vi "SomethingWith-FM.vi"() -> ()   [LabVIEW 2013]
uses:
  <vilib>/gmath/NI_Gmath.lvlib
panel:
  in  "N":dbl=1.0 caption="Numero de ciclos" format="%#_13g"
  out "mod":cluster{dbl[], dbl[]}(graph) caption="Modulação"
  out "Portadora":cluster{dbl[], dbl[]}(graph)
  out "Informação":cluster{dbl[], dbl[]}(graph)
  in  "Nc":dbl caption="Numero de amostras"
  in  "fm":dbl caption="Frequencia do sinal modulador"
  in  "fp":dbl caption="Frequencia da portadora"
  in  "E0":dbl caption="Amplitude da portadora"
  in  "Em":dbl caption="Amplitude do sinal modulador"
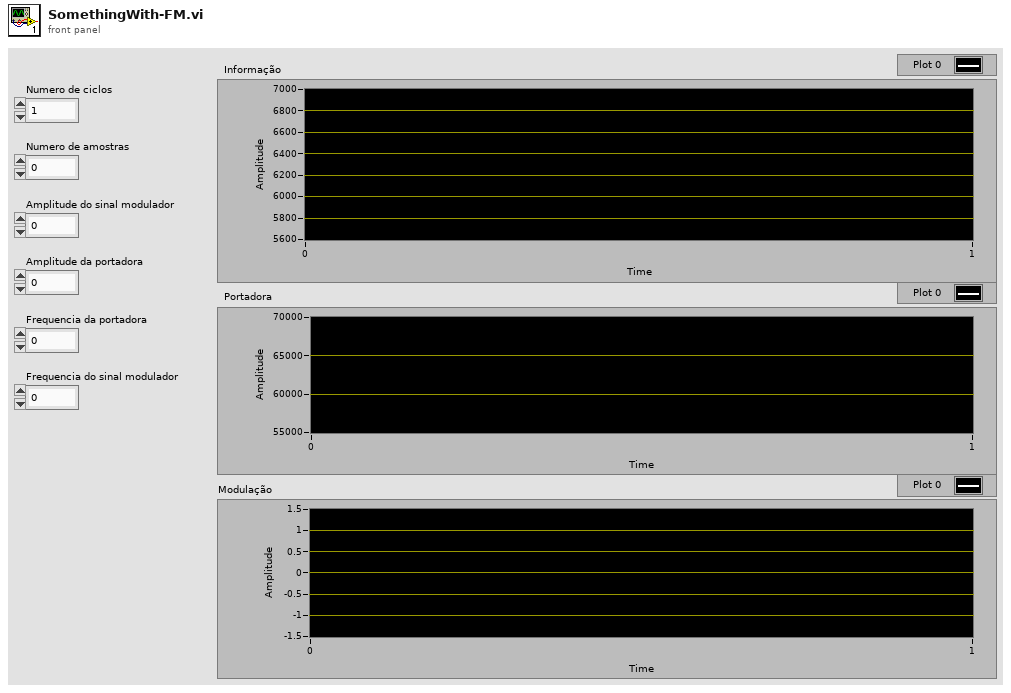
[diagram p1: front panel]
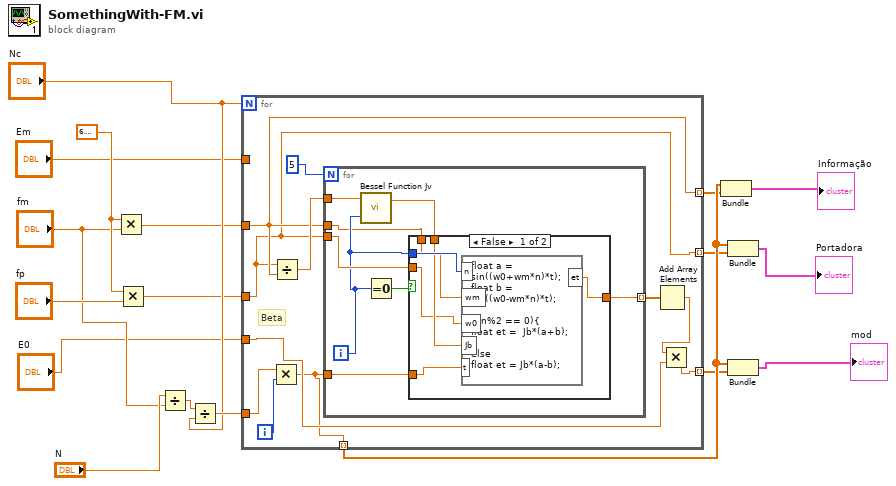
[diagram p0: block diagram]
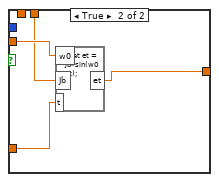
[diagram p2: hidden frame]
diagram:
  w18 = 6.283185307179586
  n1 = Multiply(x=w18, y="fm") -> (x*y=w11:dbl)
  n2 = Multiply(x=w18, y="fp") -> (x*y=w12:dbl)
  n3 = Divide(x="N", y="fm") -> (x/y=w15:dbl)
  n4 = Divide(x=w15, y="Nc") -> (x/y=w14:dbl)
  n5 = for {
    N: "Nc" -> [_]
    tunnel: "Em" -> [_]
    tunnel: "E0" -> [w22]
    tunnel: w11 -> [w24]
    tunnel: w12 -> [w23]
    tunnel: [w19] -> w9 mode=indexing
    tunnel: w14 -> [w29]
    tunnel: [w24] -> w8 mode=indexing
    tunnel: [w23] -> w7 mode=indexing
    tunnel: [w20] -> w6 mode=indexing
    i -> [w28]
    # "Beta"
    n6 = Multiply(x=w29, y=w28) -> (x*y=w19:dbl)
    n7 = Divide(x=w23, y=w24) -> (x/y=w26:dbl)
    n8 = for {
      N: 5 -> [_]
      tunnel: w26 -> [w37]
      tunnel: w23 -> [w35]
      tunnel: w19 -> [w33]
      tunnel: [w32] -> w25 mode=indexing
      tunnel: w24 -> [w30]
      i -> [w31]
      n9 = call <vilib>:"Bessel Function Jv.vi"("v"=w31, "x"=w37) -> ("Jv(x)"=w34:dbl)  [unwired: 1 in]
      n10 = Equal To 0?(x=w31) -> (x = 0?=w36:bool)
      n11 = case shown="False" w36 {
        tunnel: w35 -> [w40 w47]
        tunnel: w34 -> [w42 w46]
        tunnel: w33 -> [w41 w45]
        tunnel: [w38 w44] -> w32
        tunnel: w31 -> [w43 _]
        tunnel: w30 -> [w39 _]
        frame False {
          n12 = formula code="float a = sin((w0+wm*n)*t);\nfloat b = sin((w0-wm*n)*t);\n\nif(n%2 == 0){\nfloat et =  Jb*(a+b);\n}\nelse\nfloat et = Jb*(a-b);"("wm"=w39, "w0"=w40, "n"=w43, "Jb"=w42, "t"=w41) -> ("et"=w38:dbl)
        }
        frame True {
          n13 = formula code="float et = Jb*sin(w0*t);"("w0"=w47, "t"=w45, "Jb"=w46) -> ("et"=w44:dbl)
        }
      }
    }
    n14 = Add Array Elements(numeric array=w25) -> (sum=w21:dbl)
    n15 = Multiply(x=w21, y=w22) -> (x*y=w20:dbl)
  }
  n16 = Bundle(w9, w8) -> (→"Informação":cluster{dbl[], dbl[]})  [unwired: 1 in]
  n17 = Bundle(w9, w7) -> (→"Portadora":cluster{dbl[], dbl[]})  [unwired: 1 in]
  n18 = Bundle(w9, w6) -> (→"mod":cluster{dbl[], dbl[]})  [unwired: 1 in]
